vi "HeaderAction.vi"(0 "DefaultDevIn":refnum<class "LeafMagnetometer.lvclass"> caption="DNL_LabVIEW Object in", 11 "error in (no error)":errorcluster caption="entrée d'erreur (pas d'erreur)") -> (4 "DefaultDevOut":refnum<class "LeafMagnetometer.lvclass"> caption="DNL_LabVIEW Object out", 6 "DataNames":string[](array[string]), 8 "Instr Name":string, 10 "HeaderString":string, 15 "error out":errorcluster caption="sortie d'erreur")   [LabVIEW 2010, in "LeafMagnetometer.lvclass"]
uses:
  LeafMagnetometer.lvclass
  BaseDevice/BaseDevice.lvclass
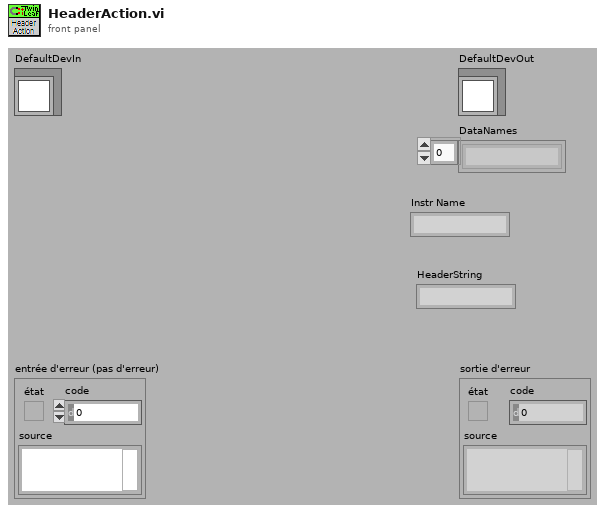
[diagram p1: front panel]
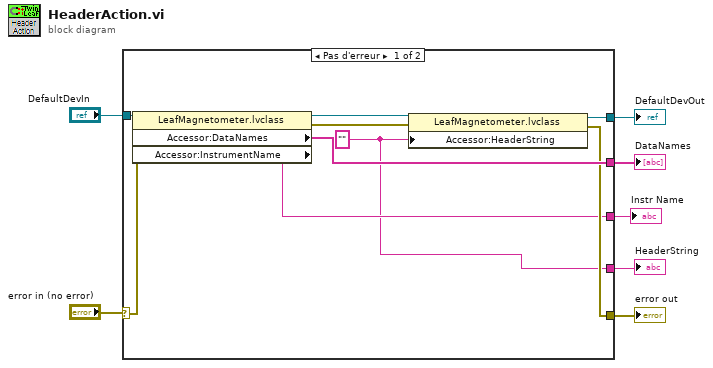
[diagram p0: block diagram]
diagram:
  n1 = case shown="Pas d'erreur" "error in (no error)" {
    selector: "error in (no error)" -> [w16 w17]
    tunnel: [w8 _] -> w6
    tunnel: [w14 _] -> w5
    tunnel: "DefaultDevIn" -> [w15 w18]
    tunnel: [w11 w17] -> w3
    tunnel: [w10 w18] -> w2
    tunnel: [w9 _] -> w1
    frame No Error {
      w8 = "" ("HeaderString")
      n2 = property class="LeafMagnetometer.lvclass"(reference=w15, error in=w16) -> (reference out=w13:refnum<class "LeafMagnetometer.lvclass">, error out=w12:errorcluster, "Accessor:DataNames"=w14:string[], "Accessor:InstrumentName"=w9:string)
      n3 = property class="LeafMagnetometer.lvclass"(reference=w13, error in=w12, "Accessor:HeaderString"=w8) -> (reference out=w10:refnum<class "LeafMagnetometer.lvclass">, error out=w11:errorcluster)
    }
    frame Error {
    }
  }
  "error out" <- w3
  "DefaultDevOut" <- w2
  "DataNames" <- w5
  "HeaderString" <- w6
  "Instr Name" <- w1
